vi "Read Allow Undefined Values.vi"(8 "error in (no error)":errorcluster, 11 "Ring.lvclass in":refnum<class "Ring.lvclass">) -> (0 "error out":errorcluster, 2 "AllowUndefVals":bool, 3 "Ring.lvclass out":refnum<class "Ring.lvclass">)   [LabVIEW 2015, in "Ring.lvclass"]
uses:
  Ring.lvclass
  Ring.lvclass/Ring.ctl
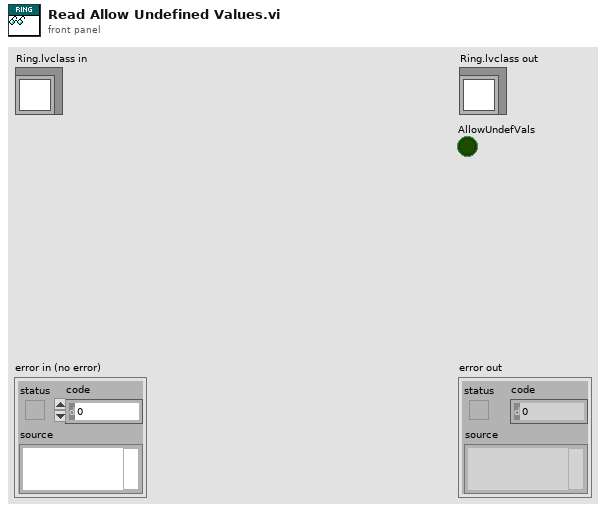
[diagram p1: front panel]
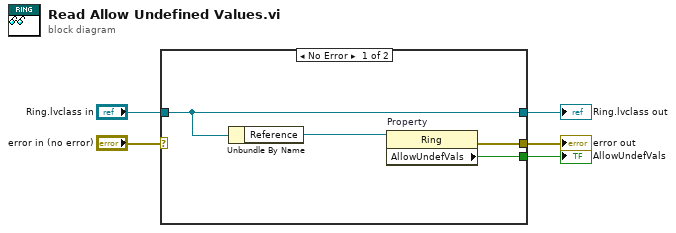
[diagram p0: block diagram]
diagram:
  n1 = case shown="No Error" "error in (no error)" {
    selector: "error in (no error)" -> [_ w11]
    tunnel: [w8 w11] -> w4
    tunnel: [w7 w10] -> w2
    tunnel: "Ring.lvclass in" -> [w7 w10]
    tunnel: [w9 _] -> w1
    frame No Error {
      n2 = Unbundle By Name(w7) -> ("Reference"=w6:refnum<vi>)
      n3 = property on="Property" class="Ring"(reference=w6) -> (error out=w8:errorcluster, "AllowUndefVals"=w9:bool)  [unwired: 1 in, 1 out]
    }
    frame Error {
    }
  }
  "error out" <- w4
  "Ring.lvclass out" <- w2
  "AllowUndefVals" <- w1
